vi "Decode Data.vi"(8 "error in (no error)":errorcluster, 9 "n character encoding":u32, 10 "Input Buffer":string) -> (0 "error out":errorcluster, 2 "Decoded Measurements":i32[](array[numeric]))   [LabVIEW 2011, in "Hokuyo URG Series.lvlib"]
doc: "This VI decodes the encoded buffers and returns an array of magnitudes.\n\nThe algorithm for decoding follows:\n1) A single data point is transmitted in three characters, so read n characters at a time\n2) Subtract 0x30 from the ascii value of each character\n3)Concatenate the n bytes to get the data point"
uses:
  Hokuyo URG Series.lvlib
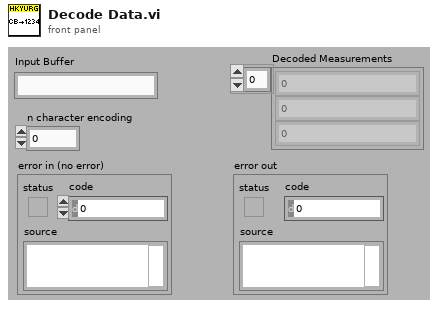
[diagram p1: front panel]
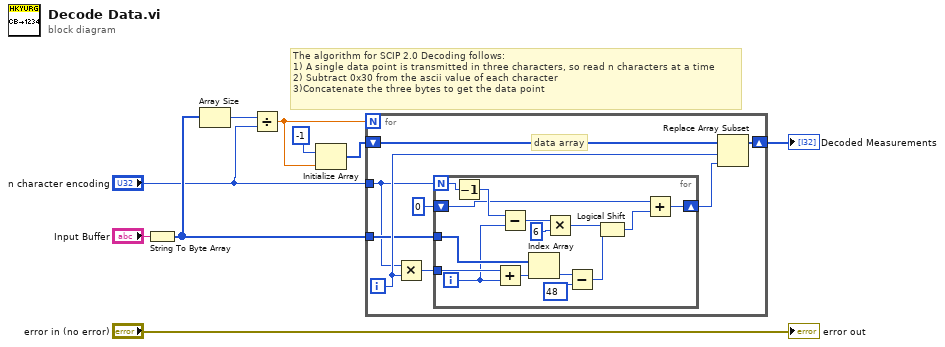
[diagram p0: block diagram]
diagram:
  # "The algorithm for SCIP 2.0 Decoding follows:\n1) A single data point is transmitted in three characters, so read n characters at a time\n2) Subtract 0x30 from the ascii value of each character\n3)Concatenate the three bytes to get the data point"
  n1 = String To Byte Array(string="Input Buffer") -> (unsigned byte array=w3:u8[])
  n2 = Array Size(array=w3) -> (size(s)=w8:i32)
  n3 = Divide(x=w8, y="n character encoding") -> (x/y=w5:dbl)
  n4 = Initialize Array(-1, w5) -> (w4:i32[])
  n5 = for {
    N: w5 -> [_]
    tunnel: w3 -> [w14]
    shift-right: [w16] -> w2
    shift-left: w4 -> [w17]
    tunnel: "n character encoding" -> [w11]
    i -> [w15]
    # "data array"
    n6 = Multiply(x=w11, y=w15) -> (x*y=w13:u32)
    n7 = for {
      N: w11 -> [w25]
      tunnel: w14 -> [w32]
      tunnel: w13 -> [w23]
      shift-right: [w27] -> w12
      shift-left: u8 0 -> [w26]
      i -> [w19]
      n8 = Decrement(x=w25) -> (x-1=w29:i32)
      n9 = Add(x=w23, y=w19) -> (x+y=w22:u32)
      n10 = Subtract(x=w29, y=w19) -> (x-y=w24:i32)
      n11 = Index Array(array=w32, index=w22) -> (element=w30:u8)
      n12 = Multiply(x=w24, y=u32 6) -> (x*y=w20:u32)
      n13 = Subtract(x=w30, y=u32 48) -> (x-y=w18:u32)
      n14 = Logical Shift(y=w20, x=w18) -> (x << y=w21:u32)
      n15 = Add(x=w26, y=w21) -> (x+y=w27:u32)
    }
    n16 = Replace Array Subset(array=w17, new element=w12, index=w15) -> (w16:i32[])
  }
  "Decoded Measurements" <- w2
  "error out" <- "error in (no error)"
